vi "Get Picture.vi"(8 "error in (no error)":errorcluster, 11 "Wood in":refnum<class "Wood.lvclass">) -> (0 "error out":errorcluster, 2 "Picture":picture, 3 "Wood out":refnum<class "Wood.lvclass">)   [LabVIEW 2020, in "Wood.lvclass"]
uses:
  Wood.lvclass
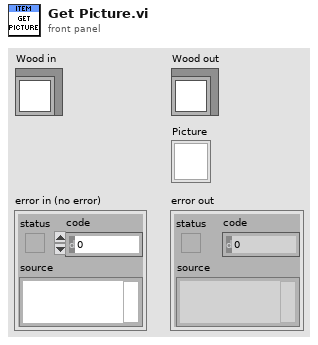
[diagram p1: front panel]
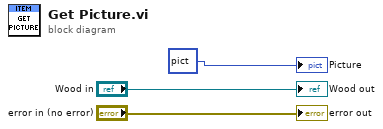
[diagram p0: block diagram]
diagram:
  "error out" <- "error in (no error)"
  "Wood out" <- "Wood in"
  "Picture" <- picture bytes[3230] ("new picture")
